vi "1B_RampAmplitude.vi"(3 "Elapsed time from Active Stim ( sec )":dbl=1.0 format="%#.3p", 4 "End-Ramp Amplitude ( mA )":dbl=5.0 format="%#.3p", 5 "Ramp Duration ( sec )":dbl=10.0 format="%#.3p") -> (0 "Expected Amplitude at time( mA )":dbl=0.5 format="%#.3p")   [LabVIEW 2010]
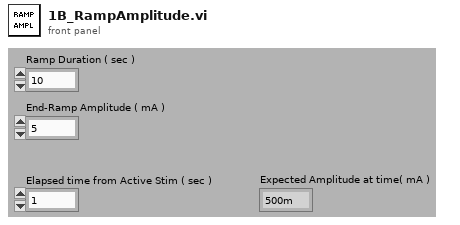
[diagram p1: front panel]
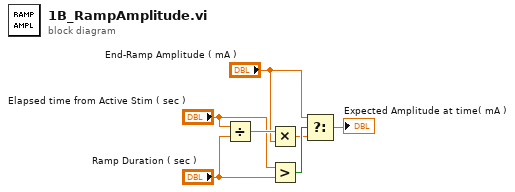
[diagram p0: block diagram]
diagram:
  n1 = Divide(x="Elapsed time from Active Stim ( sec )", y="Ramp Duration ( sec )") -> (x/y=w7:dbl)
  n2 = Multiply(x=w7, y="End-Ramp Amplitude ( mA )") -> (x*y=w1:dbl)
  n3 = Greater?(x="Elapsed time from Active Stim ( sec )", y="Ramp Duration ( sec )") -> (0:w4:bool)
  n4 = Select(t="End-Ramp Amplitude ( mA )", s=w4, f=w1) -> (s? t:f=→"Expected Amplitude at time( mA )":dbl)
